vi "Calibration.vi"(10 "Voltage":dbl[](array[numeric])=[1.3, 0.6, 0.4], 11 "Distance":dbl[](array[numeric])=[0.2, 0.5, 0.8]) -> (3 "Calibration Parameters":cluster{"m":dbl, "b":dbl, "k":dbl}={"m"=3.3068783068783096, "b"=-0.1322751322751332, "k"=0.0399999999999998})   [LabVIEW 2013]
doc: "Calculate the calibration parameters m, b and k based on a linearization method."
panel:
  # "Use this VI to calculate the Calibration Parameters of your device which are used in the Covert voltage.vi"
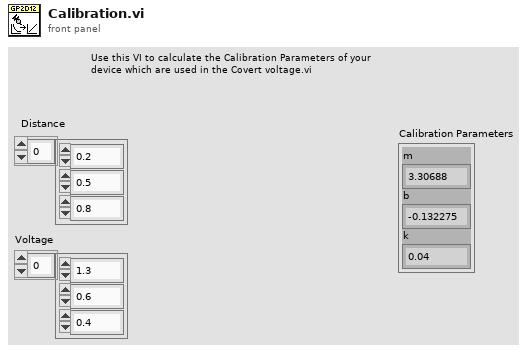
[diagram p1: front panel]
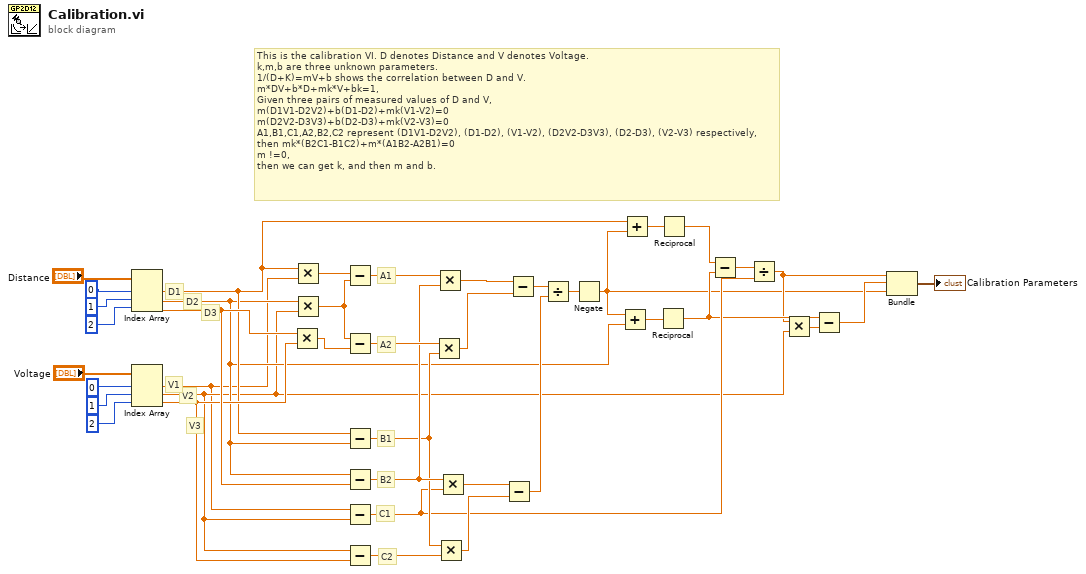
[diagram p0: block diagram]
diagram:
  # "V3"
  # "V2"
  # "D3"
  # "D2"
  # "V1"
  # "D1"
  # "This is the calibration VI. D denotes Distance and V denotes Voltage.\nk,m,b are three unknown parameters.\n1/(D+K)=mV+b shows the correlation between D and V.\nm*DV+b*D+mk*V+bk=1,\nGiven three pairs of measured values of D and V,\nm(D1V1-D2V2)+b(D1-D2)+mk(V1-V2)=0\nm(D2V2-D3V3)+b(D2-D3)+mk(V2-V3)=0\nA1,B1,C1,A2,B2,C2 represent (D1V1-D2V2), (D1-D2), (V1-V2), (D2V2-D3V3), (D2-D3), (V2-V3) respectively,\nthen mk*(B2C1-B1C2)+m*(A1B2-A2B1)=0\nm !=0,\nthen we can get k, and then m and b."
  # "C2"
  # "C1"
  # "B2"
  # "B1"
  # "A2"
  # "A1"
  n1 = Index Array(array="Distance", index #1=0 ("index"), index #2=1 ("index"), index #3=2 ("index")) -> (element #1=w17:dbl, element #2=w15:dbl, element #3=w31:dbl)
  n2 = Index Array(array="Voltage", index #1=0 ("index"), index #2=1 ("index"), index #3=2 ("index")) -> (element #1=w3:dbl, element #2=w10:dbl, element #3=w30:dbl)
  n3 = Multiply(x=w31, y=w30) -> (x*y=w1:dbl)
  n4 = Multiply(x=w17, y=w3) -> (x*y=w32:dbl)
  n5 = Multiply(x=w15, y=w10) -> (x*y=w2:dbl)
  n6 = Subtract(x=w32, y=w2) -> (x-y=w29:dbl)
  n7 = Subtract(x=w2, y=w1) -> (x-y=w28:dbl)
  n8 = Subtract(x=w17, y=w15) -> (x-y=w23:dbl)
  n9 = Subtract(x=w15, y=w31) -> (x-y=w25:dbl)
  n10 = Subtract(x=w3, y=w10) -> (x-y=w11:dbl)
  n11 = Subtract(x=w10, y=w30) -> (x-y=w24:dbl)
  n12 = Multiply(x=w28, y=w23) -> (x*y=w26:dbl)
  n13 = Multiply(x=w29, y=w25) -> (x*y=w27:dbl)
  n14 = Multiply(x=w23, y=w24) -> (x*y=w21:dbl)
  n15 = Multiply(x=w25, y=w11) -> (x*y=w22:dbl)
  n16 = Subtract(x=w22, y=w21) -> (x-y=w19:dbl)
  n17 = Subtract(x=w27, y=w26) -> (x-y=w20:dbl)
  n18 = Divide(x=w20, y=w19) -> (x/y=w18:dbl)
  n19 = Negate(x=w18) -> (-x=w5:dbl)
  n20 = Add(x=w5, y=w15) -> (x+y=w14:dbl)
  n21 = Add(x=w17, y=w5) -> (x+y=w16:dbl)
  n22 = Reciprocal(x=w14) -> (1/x=w8:dbl)
  n23 = Reciprocal(x=w16) -> (1/x=w13:dbl)
  n24 = Subtract(x=w13, y=w8) -> (x-y=w12:dbl)
  n25 = Divide(x=w12, y=w11) -> (x/y=w7:dbl)
  n26 = Multiply(x=w7, y=w10) -> (x*y=w9:dbl)
  n27 = Subtract(x=w8, y=w9) -> (x-y=w6:dbl)
  n28 = Bundle(w7, w6, w5) -> (→"Calibration Parameters":cluster{dbl, dbl, dbl})  [unwired: 1 out]
